vi "Dashboard Main.vi"() -> ()   [LabVIEW 2017]
uses:
  <vilib>/Utility/miscctls.llb/LVRowAndColumnTypeDef.ctl
  <vilib>/event_ctls.llb/eventvkey.ctl
  <vilib>/Rock Robotics/Network Tables/NT Read Numeric Array.vi
  <vilib>/Rock Robotics/WPI/Dashboard/WPI_DashboardLogging Global.vi
panel:
  out "Background 4":bool
  out "Background 3":bool
  out "Background 2":bool
  out "Background":bool
  in  "Camera Settings Right":T1={"Frame Rate"=30, "Compression"=30, "Size"=1, "DB Camera Config"=FALSE} {"Frame Rate" scale=1.0..30.0; "Compression" scale=100.0..-1.0; "Size" items=["640x480", "320x240", "160x120"]}
  in  "Camera Name Right":string(combo)="No Camera Selection"
  out "Camera Info":cluster{"Mbps LED":bool, "Mbps":dbl, "fps":dbl} {"fps" format="%#.1g"; "Mbps" format="%#.1g"}
  in  "Camera Settings":T1={"Frame Rate"=30, "Compression"=30, "Size"=1, "DB Camera Config"=FALSE} {"Frame Rate" scale=1.0..30.0; "Compression" scale=100.0..-1.0; "Size" items=["640x480", "320x240", "160x120"]}
  in  "TCP":refnum<k5>
  in  "Rec Mode":enum32{"Stop", "Record", "Playback"}(radio)
  out "Robot IP":string
  out "Image Message":string="Timeout in Camera Communications"
  in  "Dashboard Tab":T2(tab)
  out "Robot Lift Lower DIO3":bool
  out "Robot Lift Upper DIO2":bool
  out "Cube Lift DIO4":bool
  in  "Select Auto":string(combo)="Select Autonomous ..."
  out "NT Connection":bool
  out "MotorChart R":cluster{"Numeric":dbl, "Numeric":dbl}(graph)
  out "MotorChart L":cluster{"Numeric":dbl, "Numeric":dbl}(graph)
  out "MotorSliders R":cluster{"MotorSlide1":dbl, "MotorSlide2":dbl} {"MotorSlide2" scale=-1.0..1.0 scale format="%#_2e"; "MotorSlide1" scale=-1.0..1.0 scale format="%#_2e"}
  out "MotorSliders L":cluster{"MotorSlide1":dbl, "MotorSlide2":dbl} {"MotorSlide2" scale=-1.0..1.0 scale format="%#_2e"; "MotorSlide1" scale=-1.0..1.0 scale format="%#_2e"}
  out "Gyro":dbl(knob) scale=0.0..360.0
  out "JS1 Z":dbl(slide) scale=-1.0..1.0 scale format="%#_2e"
  out "JS1 Graph":cluster{"X":dbl, "Y":dbl}[](graph)
  out "JS1 Buttons":T3
  out "JS2 Z":dbl(slide) scale=-1.0..1.0 scale format="%#_2e"
  out "JS2 Graph":cluster{"X":dbl, "Y":dbl}[](graph)
  out "JS2 Buttons":T3
  out "Mode":T4(ring)=enum."Auto Disabled"
  out "Camera Image Right":T5(plugin-control)
  in  "Drive Style Selection":string(combo)="FPS"
  in  "Cube Intake Speed":dbl=10.0 min=0.0 max=10.0 step=1.0
  in  "H-Wheel":dbl=10.0 min=0.0 max=10.0 step=1.0
  in  "X-AXIS":dbl=10.0 min=0.0 max=10.0 step=1.0
  in  "Y-AXIS":dbl=10.0 min=0.0 max=10.0 step=1.0
  in  "Drive Motor Controller Selection":string(combo)="Talon SRX"
  in  "Cube Lift Down Speed":dbl=10.0 min=0.0 max=10.0 step=1.0
  in  "H-Wheel Motor Controller Selection":string(combo)="Spark"
  in  "Robot Lift Speed":dbl=10.0 min=0.0 max=10.0 step=1.0
  in  "Cube Lift Up Speed":dbl=10.0 min=0.0 max=10.0 step=1.0
  in  "MSR Slow Speed":dbl=0.5
  in  "MSR Slow Time":dbl=10.0
  in  "MSR Fast Speed":dbl=0.9
  in  "MSR Strafe Speed":dbl=0.6
  in  "MSR Fast Time":dbl=80.0
  in  "MSR Strafe Time":dbl=20.0
  in  "Move from Wall Speed":dbl=0.5
  in  "Move from Wall time":dbl=10.0
  in  "Strafe Speed":dbl=0.9
  in  "Forward Speed":dbl=0.6
  in  "Strafe Time":dbl=80.0
  in  "Forward Time":dbl=20.0
  in  "Test Slider":dbl(slide) scale=0.0..100.0 scale format="%#_3g"
  in  "On/Off":bool caption="Solenoid"
  in  "Test Name":u16(ring) items=["Select the test to run..."]
  in  "Test Tree":string(tree)
  in  "Motor":cluster{"Value":dbl, "Enable":bool} {"Value" scale=-1.0..1.0 scale format="%#_3g"}
  out "Progress":T6 {"Test Progress" scale=0.0..100.0}
  in  "Rev/Fwd":cluster{"Forward":bool, "Reverse":bool}
  in  "Test Ring":u16(ring) items=["Monochrome", "Color"]
  out "Cmd Status":string
  in  "Execute Command":bool
  in  "Command Params":string[][](table)
  in  "Command Selection":i32(listbox)
  in  "CheckList":i32(listbox)
  out "Tree":string(tree)
  out "Camera Image":T5(plugin-control)
  in  "Camera Name":string(combo)="No Camera Selection"
  # "HW"
  # "HW"
  # "Joysticks"
  # "Drive Motors"
  # "Front"
  # "Right"
  # "Left"
  # "Back"
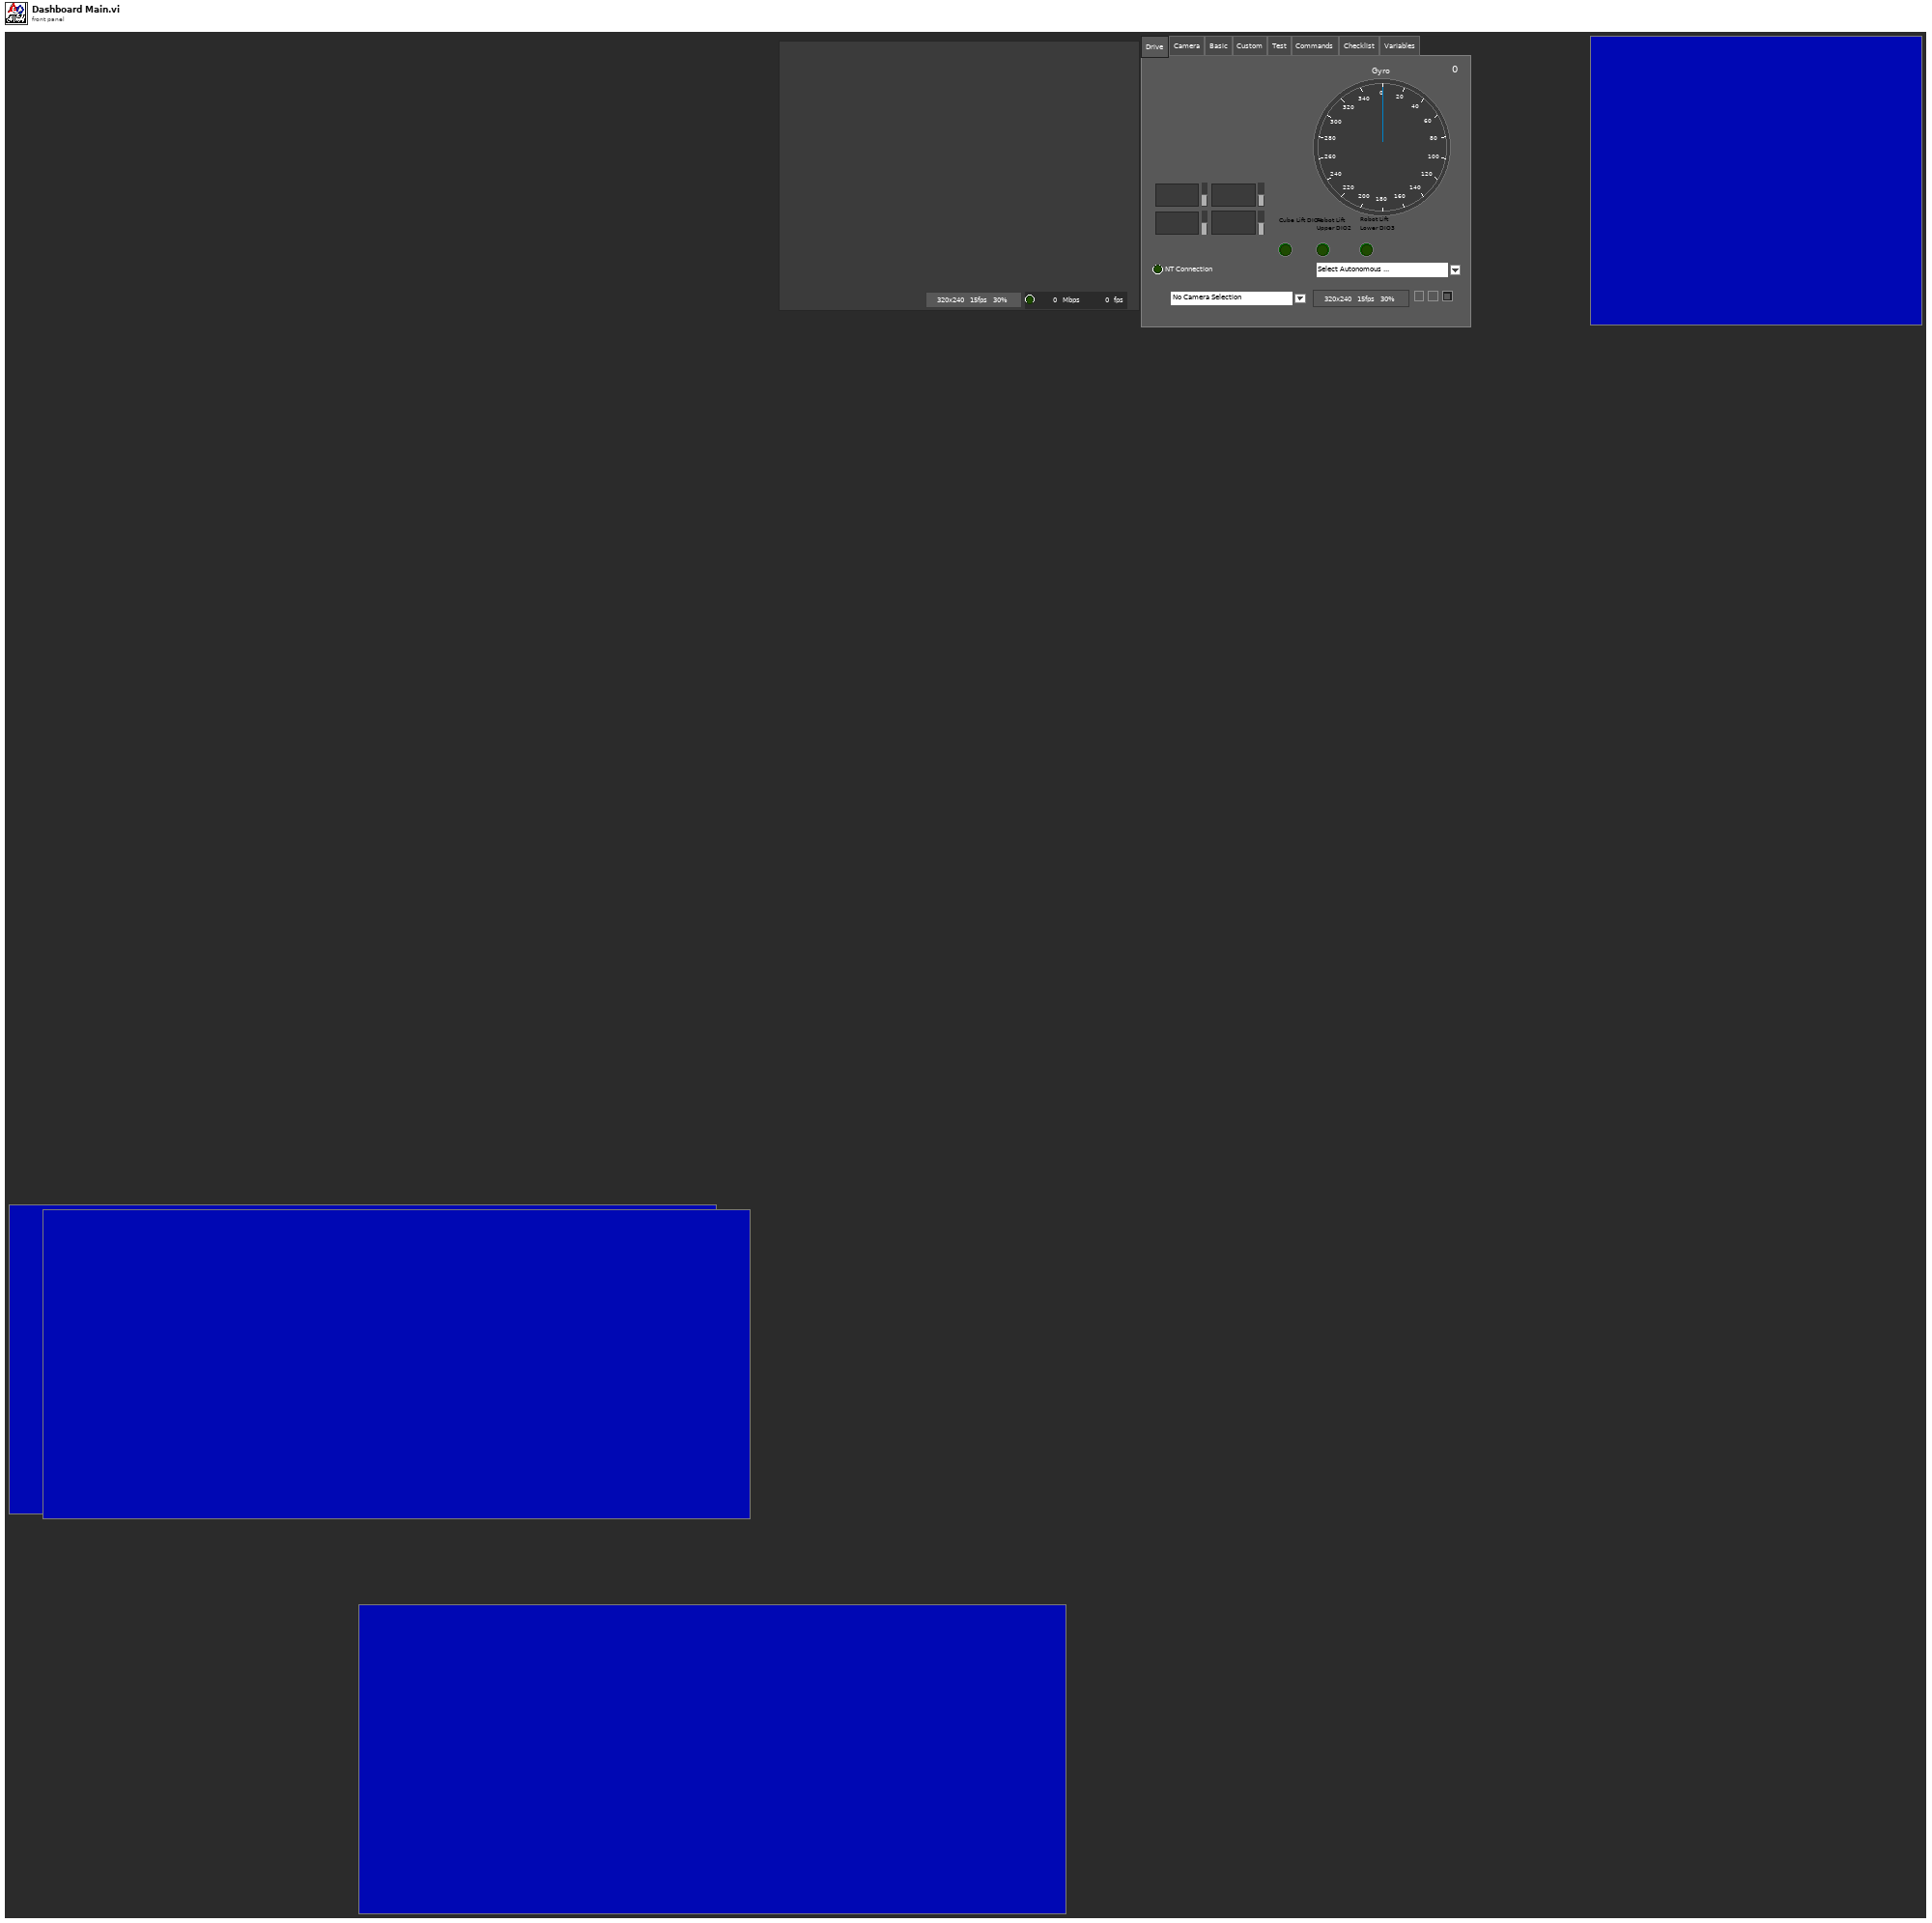
[diagram p1: front panel]
types:
  T1 = cluster{"Frame Rate":i32, "Compression":i32, "Size":u16, "DB Camera Config":bool}
  T2 = enum32{"Drive", "Camera", "Basic", "Custom", "Test", "Commands", "Checklist", "Variables"}
  T3 = cluster{bool, bool, bool, bool, bool, bool, bool, bool, bool, bool, bool, bool}
  T4 = enum8{"Tele-Op Disabled", "Tele-Op Enabled", "Auto Disabled", "Auto Enabled", "Test Disabled", "Test Enabled", "Disconnected", "No Code", "E-Stop"}
  T5 = typedef "IMAQ Image.ctl" = refnum<image>
  T6 = cluster{"Test Progress":u8, "Test Progress Text":string}
  T7 = cluster{"Save Path":path, "Interval (s)":dbl, "Keep":i32}
  T8 = typedef "Image Type" = u32
  T9 = cluster{"IDs":cluster{"RPC field ID":u16, "Unique ID":u16}, "String":string}
  T10 = cluster{"Error Strings":string, "Disable Counts":cluster{u16, u16}, "Rail Faults":cluster{u16, u16, u16}, "Robot IP":string, "DB Mode":u8, "Event Info":cluster{"Name":string, "Type":u8, "Number":u16, "Replay":u8}}
  T11 = cluster{"Storage":cluster{"Disk Free":u64, "RAM Block":u32, "RAM free":u32}, "CPU Utilization":cluster{"CPU % ISR":sgl, "CPU % Time Crit":sgl, "CPU % Timed Str":sgl, "CPU % High":sgl, "CPU % Above":sgl, "CPU % Normal":sgl, "CPU % Low":sgl}, "CAN":cluster{"% Bus Utilization":sgl, "Bus Off Cnt":u32, "TX_FIFO Full Cnt":u32, "Receive Error Cnt":u8, "Transmit Error Cnt":u8}, "HID":cluster{"HID Outputs":u32, "Rumble Low":u16, "Rumble High":u16}[]}
  T12 = cluster{"Status bits":cluster{"Test Mode":bool, "Autonomous":bool, "Enabled":bool, "Code Start":bool, "Brownout":bool, "Reserved 2":bool, "Reserved 3":bool, "E-Stop":bool}, "Code Trace":cluster{"Disabled":bool, "TeleOp":bool, "Auto":bool, "Test":bool}, "Controller Type":enum16{"unknown", "cRIO", "roboRio"}, "Code?":enum16{"unknown", "noCode", "code"}, "Battery V":dbl}
  T13 = cluster{"Control Bits":cluster{"TestMode":bool, "Autonomous":bool, "Enabled":bool, "FMS Present":bool, bool, bool, bool, "E-Stop":bool}, "Team Station ":u8, "Countdown":sgl, "Joystick Values":cluster{"Axes":dbl[], "Buttons":bool[], "POVs":i16[]}[]}
  T14 = cluster{"Axes":dbl[], "Buttons":bool[], "POVs":i16[]}[]
  T15 = cluster{"Axes":dbl[], "Buttons":bool[], "POVs":i16[]}
  T16 = cluster{"Buttons[0]":bool, "Buttons[1]":bool, "Buttons[2]":bool, "Buttons[3]":bool, "Buttons[4]":bool, "Buttons[5]":bool, "Buttons[6]":bool, "Buttons[7]":bool, "Buttons[8]":bool, "Buttons[9]":bool, "Buttons[10]":bool, "Buttons[11]":bool}
  T17 = cluster{"Camera Image":refnum<vi>, "Dashboard Tab":refnum<vi>, "Background 4":refnum<vi>, "Rec Mode":refnum<vi>, "Test Slider":refnum<vi>, "On/Off ":refnum<vi>, "Test Ring":refnum<vi>, "Rev/Fwd":refnum<vi>, "Test Name":refnum<vi>, "Motor":refnum<vi>, "Progress":refnum<vi>, "CheckList":refnum<vi>, "Tree":refnum<vi>, "Test Tree":refnum<vi>, "Command Params":refnum<vi>, "Command Selection":refnum<vi>, "Execute Command":refnum<vi>, "Cmd Status":refnum<vi>, "Camera Settings":refnum<vi>, "Camera Name":refnum<vi>, "Camera Info":refnum<vi>, "Camera Settings Right":refnum<vi>, "Camera Name Right":refnum<vi>, "Camera Image Right":refnum<vi>}
  T18 = cluster{"Camera Name":string, string, "Saved DB Images Info":cluster{"Save Path":path, "Interval (s)":dbl, "Keep":i32}}
  T19 = cluster{"Camera Name Right":string, string, "Saved DB Images Info":cluster{"Save Path":path, "Interval (s)":dbl, "Keep":i32}}
  T20 = cluster{"Operation":enum16{"Update", "Clear"}, "Color Box":u32}[]
  T21 = typedef "eventvkey.ctl" = enum16{"ASCII", "Enter", "Return", "Shift", "Ctrl", "Alt", "Cmd", "Opt", "Caps", "NumLock", "Clear", "Break", "Up", "Down", "Left", "Right", "Insert", "Delete", "Home", "End", "PageUp", "PageDown", "Escape", "Help", "Pause", "ScrollLock", "F1", "F2", "F3", "F4", "F5", "F6", "F7", "F8", "F9", "F10", "F11", "F12", "F13", "F14", "F15", "F16", "F17", "F18", "F19", "F20", "F21", "F22", "F23", "F24", "Play", "VolumeUp", "VolumeDown", "Mute", "Two Byte Char"}
  T22 = cluster{"Image Size":bool, "Image Type":bool, "Pixel Value":bool, "ROI Information":bool, "Zoom Factor":bool}
  T23 = cluster{"Operation":enum16{"Update", "Clear"}, "Color Box":u32}
  T24 = typedef "LVRowAndColumnTypeDef.ctl" = cluster{"Row":i32, "Column":i32}
  T25 = cluster{"Shift":bool, "Ctrl":bool, "Alt":bool, "Cmd":bool, "Opt":bool}
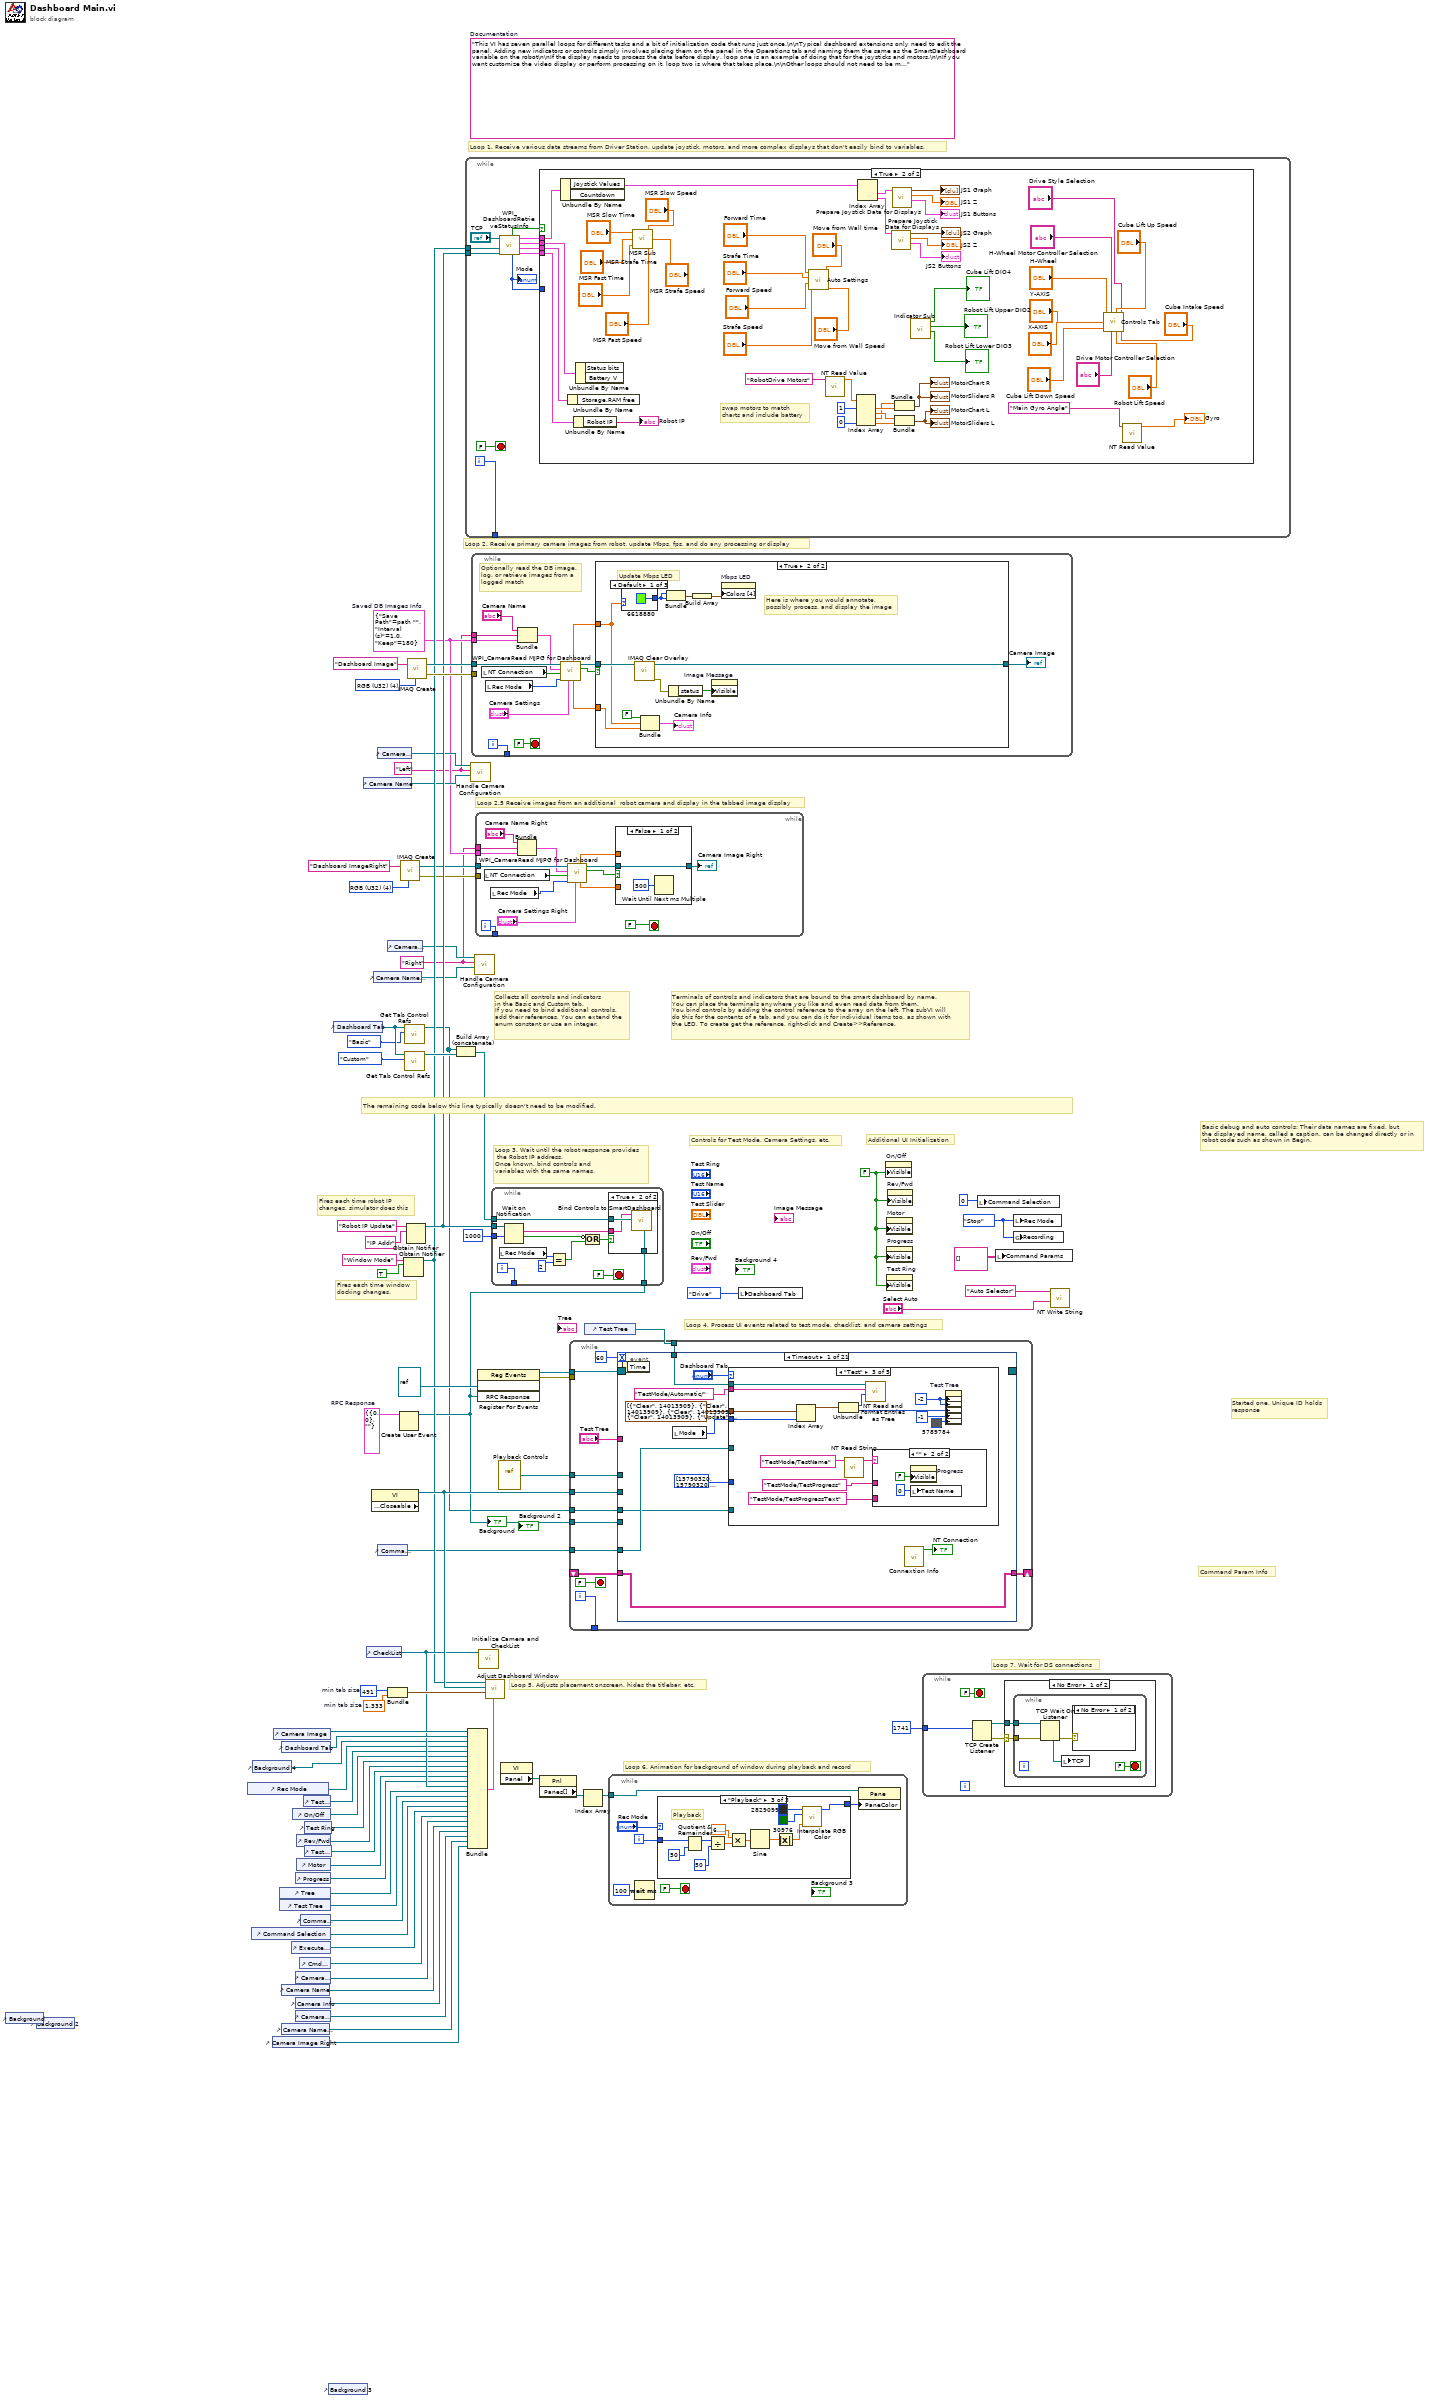
[diagram p0: block diagram]
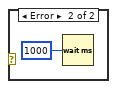
[diagram p3: hidden frame]
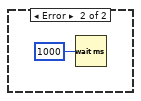
[diagram p4: hidden frame]
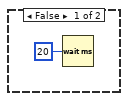
[diagram p5: hidden frame]
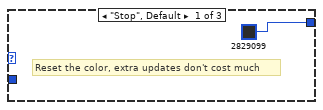
[diagram p6: hidden frame]
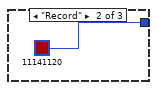
[diagram p7: hidden frame]
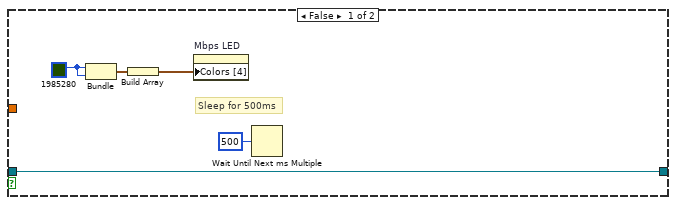
[diagram p9: hidden frame]
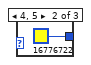
[diagram p10: hidden frame]
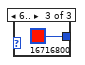
[diagram p11: hidden frame]
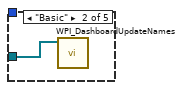
[diagram p13: hidden frame]
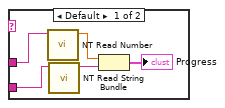
[diagram p14: hidden frame]
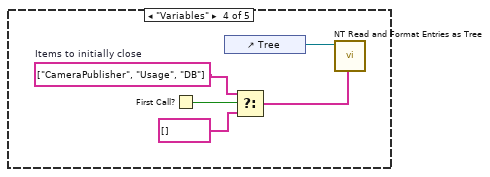
[diagram p15: hidden frame]
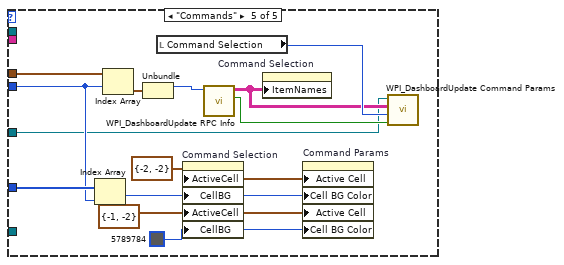
[diagram p16: hidden frame]
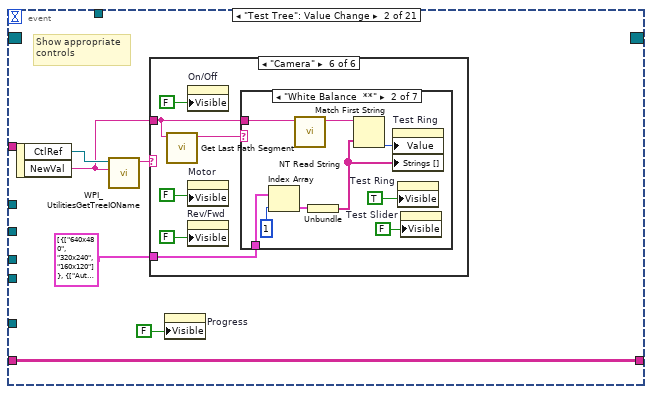
[diagram p17: hidden frame]
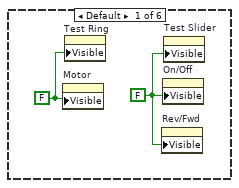
[diagram p18: hidden frame]
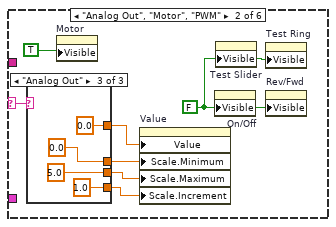
[diagram p19: hidden frame]
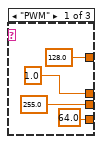
[diagram p20: hidden frame]
diagram:
  w4 = T7 {"Save Path"=path "", "Interval (s)"=1.0, "Keep"=180}  # Saved DB Images Info
  w3 = "Right"
  w2 = "Left"
  w14 = T8 4 items=["Grayscale (U8)", "Grayscale (I16)", "Grayscale (SGL)", "Complex (CSG)", "RGB (U32)", "HSL (U32)", "RGB (U64)"] ("Image Type")
  w30 = T9 {"IDs"={"RPC field ID"=0, "Unique ID"=0}, "String"=""}  # RPC Response
  w52 = 491  # min tab size
  w51 = 1.333  # min tab size
  w59 = enum32{"Stop", "Record", "Playback"}."Stop" ("Rec Mode")
  w37 = FALSE ("Visible")
  (unwired) "This VI has seven parallel loops for different tasks and a bit of initialization code that runs just once.\n\nTypical dashboard extensions only need to edit the panel. Adding new indicators or controls simply involves placing them on the panel in the Operations tab and naming them the same as the SmartDashboard variable on the robot\n\nIf the display needs to process the data before display, loop one is an example of doing that for the joysticks and motors.\n\nIf you want customize the video display or perform processing on it, loop two is where that takes place.\n\nOther loops should not need to be modified. They are pretty standard, and document the task they perform."  # Documentation
  w76 = T8 4 items=["Grayscale (U8)", "Grayscale (I16)", "Grayscale (SGL)", "Complex (CSG)", "RGB (U32)", "HSL (U32)", "RGB (U64)"] ("Image Type")
  # "Loop 2.5 Receive images from an additional  robot camera and display in the tabbed image display"
  # "Command Param Info"
  # "Started one, Unique ID holds\nresponse"
  # "Loop 7. Wait for DS connections"
  # "Basic debug and auto controls: Their data names are fixed, but\nthe displayed name, called a caption, can be changed directly or in\nrobot code such as shown in Begin."
  # "Controls for Test Mode, Camera Settings, etc."
  # "Additional UI Initialization"
  # "Loop 6. Animation for background of window during playback and record"
  # "Fires each time robot IP\nchanges, simulator does this"
  # "Fires each time window\ndocking changes."
  # "Collects all controls and indicators\nin the Basic and Custom tab.\nIf you need to bind additional controls,\nadd their references. You can extend the\nenum constant or use an integer."
  # "The remaining code below this line typically doesn't need to be modified."
  # "Loop 4. Process UI events related to test mode, checklist, and camera settings"
  # "Terminals of controls and indicators that are bound to the smart dashboard by name.\nYou can place the terminals anywhere you like and even read data from them.\nYou bind controls by adding the control reference to the array on the left. The subVI will\ndo this for the contents of a tab, and you can do it for individual items too, as shown with\nthe LED. To create get the reference, right-click and Create>>Reference."
  # "Loop 3. Wait until the robot response provides\n the Robot IP address.\nOnce known, bind controls and\nvariables with the same names."
  # "Loop 5. Adjusts placement onscreen, hides the titlebar, etc."
  # "Loop 1. Receive various data streams from Driver Station, update joystick, motors, and more complex displays that don't easily bind to variables."
  # "Loop 2. Receive primary camera images from robot, update Mbps, fps, and do any processing or display"
  n1 = control-ref of="Background"() -> ()  [unwired: 1 out]
  n2 = control-ref of="Background 2"() -> ()  [unwired: 1 out]
  n3 = control-ref of="Rec Mode"() -> (w43:refnum<vi>)
  n4 = control-ref of="Command Selection"() -> (w29:refnum<vi>)
  n5 = control-ref of="Background 4"() -> (w1:refnum<vi>)
  n6 = control-ref of="Camera Image Right"() -> (w7:refnum<vi>)
  n7 = control-ref of="Camera Image"() -> (w54:refnum<vi>)
  n8 = control-ref of="Tree"() -> (w47:refnum<vi>)
  n9 = control-ref of="Test Tree"() -> (w46:refnum<vi>)
  n10 = control-ref of="Dashboard Tab"() -> (w53:refnum<vi>)
  n11 = control-ref of="Camera Name"() -> (w20:refnum<vi>)
  n12 = control-ref of="Camera Name Right"() -> (w8:refnum<vi>)
  n13 = control-ref of="Execute Command"() -> (w31:refnum<vi>)
  n14 = control-ref of="On/Off"() -> (w41:refnum<vi>)
  n15 = control-ref of="Progress"() -> (w38:refnum<vi>)
  n16 = control-ref of="Camera Settings"() -> (w21:refnum<vi>)
  n17 = control-ref of="Camera Info"() -> (w19:refnum<vi>)
  n18 = control-ref of="Camera Settings Right"() -> (w9:refnum<vi>)
  n19 = control-ref of="Rev/Fwd"() -> (w39:refnum<vi>)
  n20 = control-ref of="Motor"() -> (w44:refnum<vi>)
  n21 = control-ref of="Cmd Status"() -> (w25:refnum<vi>)
  n22 = control-ref of="Command Params"() -> (w32:refnum<vi>)
  n23 = control-ref of="Test Slider"() -> (w42:refnum<vi>)
  n24 = control-ref of="Test Ring"() -> (w40:refnum<vi>)
  n25 = control-ref of="Test Name"() -> (w45:refnum<vi>)
  n26 = control-ref of="Background 3"() -> ()  [unwired: 1 out]
  n27 = control-ref of="Dashboard Tab"() -> (w57:refnum<vi>)
  n28 = control-ref of="Camera Name"() -> (w22:refnum<vi>)
  n29 = control-ref of="CheckList"() -> (w48:refnum<vi>)
  n30 = property class="VI" props=["Front Panel.Closeable"]() -> (reference out=w58:refnum<vi>)  [unwired: 2 in, 2 out]
  n31 = control-ref of="Camera Name Right"() -> (w10:refnum<vi>)
  n32 = control-ref of="Camera Settings"() -> (w23:refnum<vi>)
  n33 = control-ref of="Command Params"() -> (w24:refnum<vi>)
  n34 = control-ref of="Camera Settings Right"() -> (w11:refnum<vi>)
  n35 = Bundle("min tab size"=w52, "min tab size"=w51) -> (w50:cluster{"min tab size":i32, "min tab size":dbl})  [unwired: 1 in]
  n36 = Create User Event(user event datatype=w30) -> (user event=w26:refnum<user-event>)  [unwired: 1 in, 1 out]
  n37 = call "IMAQ Create"("Image Name"="Dashboard ImageRight", "Image Type"=w14) -> ("New Image"=w13:T5, "error out"=w12:errorcluster)  [unwired: 2 in, 1 out]
  n38 = Obtain Notifier(name (unnamed)="Window Mode", notification data type=TRUE) -> (notifier out=w35:refnum<notifier>)  [unwired: 2 in, 2 out]
  n39 = call <vilib>:"Get Tab Control Refs.vi"("Page Index"=T2."Basic" ("Dashboard Tab"), "TabControl in"=w57) -> ("ControlsOnPage"=w18:refnum<vi>[])  [unwired: 9 in]
  n40 = call <vilib>:"Get Tab Control Refs.vi"("Page Index"=T2."Custom" ("Dashboard Tab"), "TabControl in"=w57) -> ("ControlsOnPage"=w56:refnum<vi>[])  [unwired: 9 in]
  n41 = Obtain Notifier(name (unnamed)="Robot IP Update", notification data type="IP Addr" ("name (unnamed)")) -> (notifier out=w36:refnum<notifier>)  [unwired: 2 in, 2 out]
  n42 = call "IMAQ Create"("Image Name"="Dashboard Image", "Image Type"=w76) -> ("New Image"=w74:T5, "error out"=w73:errorcluster)  [unwired: 2 in, 1 out]
  n43 = Build Array (concatenate)(w18, w56) -> (w55:refnum<vi>[])
  n44 = while {
    tunnel: [w86] -> _
    tunnel: w36 -> [w80]
    tunnel: w35 -> [w77]
    i -> [w86]
    stop <- FALSE stop-if-true
    n45 = call <vilib>:"WPI_DashboardRetrieveStatusInfo.vi"("Binding Refnum"=w80, "Window Mode Notifier"=w77, "TCP Cnx"="TCP") -> ("Power and Errors"=w81:T10, "Robot Metrics"=w84:T11, "Status Info"=w85:T12, "Control Info"=w82:T13, "Robot Mode"=w79:T4, "Process?"=w83:bool)  [unwired: 3 in]
    "Mode" <- w79
    n46 = case shown="True" w83 {
      tunnel: w85 -> [_ w139]
      tunnel: w84 -> [_ w138]
      tunnel: w82 -> [_ w137]
      tunnel: w81 -> [_ w136]
      tunnel: w79 -> [_ _]
      frame False {
        n47 = Wait (ms)(milliseconds to wait=u32 20) -> ()  [unwired: 1 out]
      }
      frame True {
        # "swap motors to match\ncharts and include battery"
        n48 = Unbundle By Name(w137) -> ("Joystick Values"=w127:T14)  [unwired: 1 out]
        n49 = Unbundle By Name(w138) -> ()  [unwired: 1 out]
        n50 = Unbundle By Name(w136) -> ("Robot IP"=→"Robot IP":string)
        n51 = Unbundle By Name(w139) -> ()  [unwired: 2 out]
        n52 = call "MSR Sub.vi"("MSR Fast Speed"="MSR Fast Speed", "MSR Strafe Speed"="MSR Strafe Speed", "MSR Slow Speed"="MSR Slow Speed", "MSR Fast Time"="MSR Fast Time", "MSR Strafe Time"="MSR Strafe Time", "MSR Slow Time"="MSR Slow Time") -> ()
        n53 = call "Auto Settings.vi"("Mid Switch Forward Time"="Forward Time", "Mid Switch Strafe Time"="Strafe Time", "Mid Switch Forward Speed"="Forward Speed", "Mid Switch Strafe Speed"="Strafe Speed", "Strafe From Wall Time"="Move from Wall time", "Strafe From Wall Speed"="Move from Wall Speed") -> ()  [unwired: 5 in]
        n54 = call-poly <vilib>:"NT Read Value.vi"("Name"="RobotDrive Motors") -> ("Numeric Array"=w117:dbl[])  [unwired: 9 in, 1 out]
        n55 = Index Array(array=w117, index #1=1, index #4=0) -> (element #1=w131:dbl, element #2=w132:dbl, element #3=w130:dbl, element #4=w135:dbl)  [unwired: 2 in]
        n56 = Index Array(array=w127) -> (element #1=w126:T15, element #2=w122:T15)  [unwired: 2 in]
        n57 = call "Prepare Joystick Data for Displays.vi"("Joystick Values"=w122) -> ("Buttons"=→"JS2 Buttons":T16, "Z Axis"=→"JS2 Z":dbl, "Cartesian Data"=→"JS2 Graph":cluster{"X axis":dbl, "X axis":dbl}[])  [unwired: 8 in]
        n58 = call "Prepare Joystick Data for Displays.vi"("Joystick Values"=w126) -> ("Buttons"=→"JS1 Buttons":T16, "Z Axis"=→"JS1 Z":dbl, "Cartesian Data"=→"JS1 Graph":cluster{"X axis":dbl, "X axis":dbl}[])  [unwired: 8 in]
        n59 = Bundle("Numeric"=w130, "Numeric"=w131) -> (→"MotorChart R" →"MotorSliders R":cluster{"Numeric":dbl, "Numeric":dbl})  [unwired: 1 in]
        n60 = Bundle("Numeric"=w132, "Numeric"=w135) -> (→"MotorChart L" →"MotorSliders L":cluster{"Numeric":dbl, "Numeric":dbl})  [unwired: 1 in]
        n61 = call "Indicator Sub.vi"() -> ("Robot Lift Lower"=→"Robot Lift Lower DIO3":bool, "Robot Lift Upper"=→"Robot Lift Upper DIO2":bool, "Cube Lift"=→"Cube Lift DIO4":bool)  [unwired: 9 in]
        n62 = call "Controls Tab.vi"("H-Wheel"="H-Wheel", "H-Wheel Motor Controller Selection"="H-Wheel Motor Controller Selection", "Y-AXIS"="Y-AXIS", "Cube Lift Down Motor"="Cube Lift Down Speed", "Motor Controller Selection"="Drive Motor Controller Selection", "Cube Lift Up Motor"="Cube Lift Up Speed", "Drive Style Selection"="Drive Style Selection", "X-AXIS"="X-AXIS", "Robot Lift Motor"="Robot Lift Speed", "Cube Intake Motor"="Cube Intake Speed") -> ()
        n63 = call-poly <vilib>:"NT Read Value.vi"("Name"="Main Gyro Angle") -> ("Numeric"=→"Gyro":dbl)  [unwired: 9 in, 1 out]
      }
    }
  }
  n64 = Bundle("Camera Image"=w54, "Dashboard Tab"=w53, "Background 4"=w1, "Rec Mode"=w43, "Test Slider"=w42, "On/Off"=w41, "Test Ring"=w40, "Rev/Fwd"=w39, "Test Name"=w45, "Motor"=w44, "Progress"=w38, "CheckList"=w48, "Tree"=w47, "Test Tree"=w46, "Command Params"=w32, "Command Selection"=w29, "Execute Command"=w31, "Cmd Status"=w25, "Camera Settings"=w21, "Camera Name"=w20, "Camera Info"=w19, "Camera Settings Right"=w9, "Camera Name Right"=w8, "Camera Image Right"=w7) -> (w49:T17)  [unwired: 1 in]
  n65 = call "Handle Camera Configuration.vi"("CameraNameRef"=w22, "Display Name"=w2, "ClusterRef"=w23) -> ()  [unwired: 9 in]
  n66 = while {
    tunnel: w74 -> [w152]
    tunnel: w73 -> [_]
    tunnel: [w153] -> _
    tunnel: w4 -> [w143]
    tunnel: w2 -> [w140]
    i -> [w153]
    stop <- FALSE stop-if-true
    # "Optionally read the DB image,\nlog, or retrieve images from a\nlogged match"
    n67 = local read "NT Connection"() -> (w144:bool)
    n68 = local read "Rec Mode"() -> (w148:enum32{"Stop", "Record", "Playback"})
    n69 = Bundle("Camera Name"="Camera Name", w140, "Saved DB Images Info"=w143) -> (w142:T18)  [unwired: 1 in]
    n70 = call <vilib>:"WPI_CameraRead MJPG for Dashboard.vi"("Camera Settings"="Camera Settings", "Rec Mode"=w148, "NT Connection"=w144, "Capture Info"=w142, "Refnum in"=w152) -> ("Active"=w150:bool, "Refnum out"=w151:T5, "FPS"=w149:dbl, "Bandwidth (Mbps)"=w147:dbl)  [unwired: 3 in]
    n71 = case shown="True" w150 {
      tunnel: w151 -> [w155 w166]
      tunnel: w147 -> [_ w163]
      tunnel: w149 -> [_ w164]
      tunnel: [w155 w160] -> w145
      frame False {
        w157 = u32 1985280 ("Color Box")
        # "Sleep for 500ms"
        n72 = Bundle("Color Box"=w157, "Color Box"=w157) -> (w158:cluster{"Color Box":u32, "Color Box":u32})  [unwired: 1 out]
        n73 = Build Array(w158) -> (w156:cluster{"Color Box":u32, "Color Box":u32}[])
        n74 = property on="Mbps LED" class="Bool (strict)"("Colors [4]"=w156) -> ()  [unwired: 2 in, 2 out]
        n75 = Wait Until Next ms Multiple(millisecond multiple=u32 500) -> ()  [unwired: 1 out]
      }
      frame True {
        # "Here is where you would annotate,\npossibly process, and display the image"
        # "Update Mbps LED"
        n76 = case shown="Default" w163 {
          tunnel: [u32 6618880 ("Color Box") u32 16776722 ("Color Box") u32 16716800 ("Color Box")] -> w167
          frame Default {
          }
          frame 4, 5 {
          }
          frame 6.. {
          }
        }
        n77 = call "IMAQ Clear Overlay"("Image"=w166) -> ("error out"=w169:errorcluster, "Image Out"=w160:T5)  [unwired: 2 in, 7 out]
        n78 = Bundle(FALSE, "Bandwidth (Mbps)"=w163, "FPS"=w164) -> (→"Camera Info":cluster{bool, "Bandwidth (Mbps)":dbl, "FPS":dbl})  [unwired: 1 in]
        n79 = Bundle("Color Box"=w167, "Color Box"=w167) -> (w168:cluster{"Color Box":u32, "Color Box":u32})  [unwired: 1 out]
        n80 = Unbundle By Name(w169) -> ("status"=w170:bool)
        n81 = Build Array(w168) -> (w165:cluster{"Color Box":u32, "Color Box":u32}[])
        n82 = property on="Image Message" class="Str"("Visible"=w170) -> ()  [unwired: 2 in, 2 out]
        n83 = property on="Mbps LED" class="Bool (strict)"("Colors [4]"=w165) -> ()  [unwired: 2 in, 2 out]
      }
    }
    "Camera Image" <- w145
  }
  n84 = call "Handle Camera Configuration.vi"("CameraNameRef"=w10, "Display Name"=w3, "ClusterRef"=w11) -> ()  [unwired: 9 in]
  n85 = while {
    tunnel: w13 -> [w188]
    tunnel: w12 -> [_]
    tunnel: [w183] -> _
    tunnel: w4 -> [w177]
    tunnel: w3 -> [w174]
    i -> [w183]
    stop <- FALSE stop-if-true
    n86 = local read "NT Connection"() -> (w178:bool)
    n87 = local read "Rec Mode"() -> (w187:enum32{"Stop", "Record", "Playback"})
    n88 = Bundle("Camera Name Right"="Camera Name Right", w174, "Saved DB Images Info"=w177) -> (w176:T19)  [unwired: 1 in]
    n89 = call <vilib>:"WPI_CameraRead MJPG for Dashboard.vi"("Camera Settings"="Camera Settings Right", "Rec Mode"=w187, "NT Connection"=w178, "Capture Info"=w176, "Refnum in"=w188) -> ("Active"=w182:bool, "Refnum out"=w185:T5, "FPS"=w180:dbl, "Bandwidth (Mbps)"=w181:dbl)  [unwired: 3 in]
    n90 = case shown="False" w182 {
      tunnel: w185 -> [w189 w191]
      tunnel: w181 -> [_ _]
      tunnel: w180 -> [_ _]
      tunnel: [w189 w191] -> w179
      frame False {
        n91 = Wait Until Next ms Multiple(millisecond multiple=u32 500) -> ()  [unwired: 1 out]
      }
      frame True {
      }
    }
    "Camera Image Right" <- w179
  }
  n92 = register-events(refnum<vi> refnum, w26) -> (reference out=w63:refnum<event-registration>, error out=w62:errorcluster)  [unwired: 2 in]
  n93 = call "Initialize Camera and CheckList.vi"("ListBox in"=w48) -> ()  [unwired: 11 in]
  n94 = call "Adjust Dashboard Window.vi"("Sizing Refnums"=w49, "Size Constraints"=w50, "VI"=w58, "WIn Mode"=w35) -> ()  [unwired: 8 in]
  n95 = while {
    tunnel: w55 -> [w203]
    tunnel: w36 -> [w201]
    tunnel: [w199] -> _
    tunnel: u32 1000 ("milliseconds to wait") -> [w198]
    tunnel: w26 -> [w192]
    i -> [w199]
    stop <- FALSE stop-if-true
    n96 = local read "Rec Mode"() -> (w194:enum32{"Stop", "Record", "Playback"})
    n97 = Wait on Notification(notifier=w201, timeout in ms (-1)=w198) -> (notification=w200:string, timed out?=w196:bool)  [unwired: 2 in, 2 out]
    n98 = Equal?(x=w194, y=u16 2 ("Rec Mode")) -> (x = y?=w195:bool)
    n99 = Compound Arithmetic op=OR(invert w196, w195) -> (w197:bool)
    n100 = case shown="True" w197 {
      tunnel: w203 -> [_ w206]
      tunnel: w200 -> [_ w205]
      tunnel: w192 -> [_ w204]
      frame False {
      }
      frame True {
        n101 = call <vilib>:"Bind Controls to SmartDashboard.vi"("RPC ref"=w204, "Bound Control Refs"=w206, "Server IP Address"=w205) -> ()  [unwired: 9 in]
      }
    }
  }
  n102 = vi-ref "Playback Controls.vi"() -> (w64:refnum<vi>)
  n103 = property class="VI"() -> ("Panel"=w66:refnum<vi>)  [unwired: 2 in, 2 out]
  n104 = property class="Pnl"(reference=w66) -> ("Panes[]"=w67:refnum<vi>[])  [unwired: 1 in, 2 out]
  n105 = Index Array(array=w67) -> (element=w65:refnum<vi>)  [unwired: 1 in]
  n106 = control-ref of="Test Tree"() -> (w68:refnum<vi>)
  n107 = while {
    tunnel: [w216] -> _
    tunnel: w68 -> [w215]
    tunnel: w64 -> [w214]
    tunnel: w63 -> [w213]
    tunnel: w62 -> [_]
    tunnel: w58 -> [w212]
    tunnel: w26 -> [w211]
    tunnel: w24 -> [w210]
    shift-right: [w209] -> _
    shift-left: _ -> [w208]
    tunnel: w18 -> [w207]
    i -> [w216]
    stop <- FALSE stop-if-true
    n108 = event shown="[0] Timeout" {
      selector: w213 -> [_ _ _ _ _ _ _ _ _ _ _ _ _ _ _ _ _ _ _ _ _]
      dyn-events: [_ _ _ _ _ _ _ _ _ _ _ _ _ _ _ _ w476 _ _ _ _] -> _
      timeout: u32 60 ("milliseconds to wait") -> [_ _ _ _ _ _ _ _ _ _ _ _ _ _ _ _ _ _ _ _ _]
      tunnel: w215 -> [w228 _ _ _ _ _ _ _ _ _ _ _ _ _ _ _ _ _ _ _ _]
      tunnel: "Test Tree" -> [_ _ _ _ _ _ _ _ _ _ _ w443 w451 w453 w457 w465 _ _ _ _ _]
      tunnel: w214 -> [_ _ _ _ _ _ _ _ _ _ _ _ _ _ _ _ w478 _ w496 _ _]
      tunnel: w212 -> [_ _ _ _ _ _ _ _ _ _ _ _ _ _ _ _ w474 _ _ _ _]
      tunnel: w211 -> [_ _ _ _ _ _ _ _ _ _ _ _ _ _ _ _ w472 _ _ _ _]
      tunnel: w210 -> [w223 _ _ _ _ _ w394 _ _ _ _ _ _ _ _ _ _ _ _ _ _]
      tunnel: [w222 w271 w373 w378 w387 w391 w392 w401 w411 w418 w430 w442 w449 w452 w456 w464 w471 w491 w493 w497 w510] -> w209
      tunnel: w208 -> [w222 w271 w373 w378 w387 w391 w392 _ _ w418 w430 w442 w449 w452 w456 w464 w471 w491 w493 w497 w510]
      tunnel: w207 -> [w220 _ _ _ _ _ _ _ _ _ _ _ _ _ _ _ _ _ _ _ _]
      event Timeout {
        n109 = event-data() -> ()  [unwired: 1 in, 1 out]
        n110 = local read "Mode"() -> (w225:T4)
        n111 = case shown="\"Test\"" "Dashboard Tab" {
          tunnel: w228 -> [_ _ w244 _ _]
          tunnel: "TestMode/Automatic/" ("Name Pattern") -> [_ _ w243 _ _]
          tunnel: T20 [{"Operation"=enum."Clear", "Color Box"=14013909}, {"Operation"=enum."Clear", "Color Box"=14013909}, {"Operation"=enum."Clear", "Color Box"=14013909}, {"Operation"=enum."Clear", "Color Box"=14013909}, {"Operation"=enum."Update", "Color Box"=14013909}, {"Operation"=enum."Update", "Color Box"=16777215}, {"Operation"=enum."Clear", "Color Box"=14013909}, {"Operation"=enum."Clear", "Color Box"=14013909}, {"Operation"=enum."Clear", "Color Box"=14013909}] -> [_ _ w236 _ w264]
          tunnel: w225 -> [_ _ w235 _ w263]
          tunnel: u32[] [15790320, 15790320, 15790320, 15790320, 16777215, 16777215, 15790320, 15790320, 15790320] -> [_ _ _ _ w269]
          tunnel: w223 -> [_ _ _ _ w257]
          tunnel: w220 -> [_ w230 _ _ _]
          frame "Custom", Default {
          }
          frame "Basic" {
            n112 = call <vilib>:"WPI_DashboardUpdateNames.vi"("Controls on Tab"=w230) -> ()  [unwired: 11 in]
          }
          frame "Test" {
            w242 = -2 ("Active Item:Row Number")
            n113 = Index Array(array=w236, index=w235) -> (element=w237:T23)
            n114 = Unbundle(w237) -> ("Operation"=w238:enum16{"Update", "Clear"}, "Color Box"=w239:u32)
            n115 = call <vilib>:"NT Read String.vi"("Name"="TestMode/TestName") -> ("String"=w233:string)  [unwired: 9 in, 1 out]
            n116 = call <vilib>:"NT Read and Format Entries as Tree.vi"("Operation"=w238, "Name Pattern"=w243, "Tree Refnum"=w244) -> ()  [unwired: 7 in, 2 out]
            n117 = case shown="\"\"" w233 {
              tunnel: "TestMode/TestProgress" ("Name") -> [w246 _]
              tunnel: "TestMode/TestProgressText" ("Name") -> [w245 _]
              frame Default {
                n118 = call <vilib>:"NT Read Number.vi"("Name"=w246) -> ("Numeric"=w247:dbl)  [unwired: 9 in, 1 out]
                n119 = call <vilib>:"NT Read String.vi"("Name"=w245) -> ("String"=w248:string)  [unwired: 9 in, 1 out]
                n120 = Bundle("Numeric"=w247, "String"=w248) -> (→"Progress":cluster{"Numeric":dbl, "String":string})  [unwired: 1 in]
              }
              frame "" {
                n121 = property on="Progress" class="Clust (strict)"("Visible"=FALSE) -> ()  [unwired: 2 in, 2 out]
                n122 = local write "Test Name"(u16 0) -> ()
              }
            }
            n123 = property on="Test Tree" class="Tree (strict)"("Active Item Row Number"=w242, "ActiveColNum"=w242, "CellBG"=w239, "Active Item Row Number"=-1 ("Active Item:Row Number"), "CellBG"=u32 5789784 ("Color Box")) -> ()  [unwired: 2 in, 2 out]
          }
          frame "Variables" {
            w254 = string[] ["CameraPublisher", "Usage", "DB"]  # Items to initially close
            n124 = First Call?() -> (First Call?: T/F=w255:bool)
            n125 = control-ref of="Tree"() -> (w256:refnum<vi>)
            n126 = Select(t=w254, s=w255, f=string[] []) -> (s? t:f=w252:string[])
            n127 = call <vilib>:"NT Read and Format Entries as Tree.vi"("Tags to  Close"=w252, "Tree Refnum"=w256) -> ()  [unwired: 8 in, 2 out]
          }
          frame "Commands" {
            w265 = u32 5789784 ("Color Box")
            w266 = T24 {"Row"=-1, "Column"=-2} ("Active Cell:Active Cell")
            w268 = T24 {"Row"=-2, "Column"=-2} ("Active Cell:Active Cell")
            n128 = Index Array(array=w269, index=w263) -> (element=w267:u32)
            n129 = Index Array(array=w264, index=w263) -> (element=w262:T23)
            n130 = Unbundle(w262) -> ("Operation"=w261:enum16{"Update", "Clear"})  [unwired: 1 out]
            n131 = local read "Command Selection"() -> (w260:i32)
            n132 = property on="Command Selection" class="MCListbox (strict)"("ActiveCell"=w268, "CellBG"=w267, "ActiveCell"=w266, "CellBG"=w265) -> ()  [unwired: 2 in, 2 out]
            n133 = call <vilib>:"WPI_DashboardUpdate RPC Info.vi"("Operation"=w261) -> ("update"=w259:bool, "commands"=w258:string[][])  [unwired: 9 in]
            n134 = property on="Command Selection" class="MCListbox (strict)"("ItemNames"=w258) -> ()  [unwired: 2 in, 2 out]
            n135 = property on="Command Params" class="Tbl (strict)"("Active Cell"=w268, "Cell BG Color"=w267, "Active Cell"=w266, "Cell BG Color"=w265) -> ()  [unwired: 2 in, 2 out]
            n136 = call <vilib>:"WPI_DashboardUpdate Command Params.vi"("Update"=w259, "NewVal"=w260, "Commands"=w258, "Param Tbl"=w257) -> ()  [unwired: 7 in, 1 out]
          }
        }
        n137 = call <vilib>:"Connextion Info.vi"() -> ("Connected"=→"NT Connection":bool)  [unwired: 10 in, 1 out]
      }
      event "Test Tree": Value Change {
        # "Show appropriate\ncontrols"
        n138 = event-data() -> ("CtlRef"=w274:refnum<vi>, "NewVal"=w272:string)  [unwired: 1 in]
        n139 = call <vilib>:"WPI_UtilitiesGetTreeIOName.vi"("NewVal"=w272, "TreeControl in"=w274) -> ("I/O Name"=w275:string)  [unwired: 9 in]
        n140 = case shown="\"Camera\"" w275 {
          selector: w275 -> [_ w282 _ w304 w313 _]
          tunnel: w272 -> [_ _ w301 w303 _ w320]
          tunnel: cluster{string[]}[] [{["640x480", "320x240", "160x120"]}, {["Auto", "Fixed indoor", "Fixed outdoor 1", "Fixed outdoor 2", "Fixed fluorescent 1", "Fixed fluorescent 2", "Hold current"]}, {["Auto", "Flicker-free 50 Hz", "Flicker-free 60 Hz", "Hold current"]}, {["None", "Prioritize frame rate", "Prioritize image quality"]}, {["Monochrome", "Color"]}] -> [_ _ _ _ _ w319]
          frame Default {
            w277 = FALSE ("Visible")
            w276 = FALSE ("Visible")
            n141 = property on="Motor" class="Clust (strict)"("Visible"=w276) -> ()  [unwired: 2 in, 2 out]
            n142 = property on="Test Ring" class="Ring (strict)"("Visible"=w276) -> ()  [unwired: 2 in, 2 out]
            n143 = property on="Rev/Fwd" class="Clust (strict)"("Visible"=w277) -> ()  [unwired: 2 in, 2 out]
            n144 = property on="On/Off" class="Bool (strict)"("Visible"=w277) -> ()  [unwired: 2 in, 2 out]
            n145 = property on="Test Slider" class="Slide (strict)"("Visible"=w277) -> ()  [unwired: 2 in, 2 out]
          }
          frame "Analog Out", "Motor", "PWM" {
            w283 = FALSE ("Visible")
            n146 = case shown="\"Analog Out\"" w282 {
              tunnel: [1.0 ("Value") -1.0 ("Value") 0.0 ("Value")] -> w281
              tunnel: [255.0 ("Value") 1.0 ("Value") 5.0 ("Value")] -> w280
              tunnel: [128.0 ("Value") 0.0 ("Value") 0.0 ("Value")] -> w279
              tunnel: [64.0 ("Value") 0.5 ("Value") 1.0 ("Value")] -> w278
              frame "PWM" {
              }
              frame "Motor", Default {
              }
              frame "Analog Out" {
              }
            }
            n147 = property on="Motor" class="Clust (strict)"("Visible"=TRUE) -> ()  [unwired: 2 in, 2 out]
            n148 = property on="Value" class="Slide (strict)"("Value"=w279, "Scale.Minimum"=w281, "Scale.Maximum"=w280, "Scale.Increment"=w278) -> ()  [unwired: 2 in, 2 out]
            n149 = property on="On/Off" class="Bool (strict)"("Visible"=w283) -> ()  [unwired: 2 in, 2 out]
            n150 = property on="Test Slider" class="Slide (strict)"("Visible"=w283) -> ()  [unwired: 2 in, 2 out]
            n151 = property on="Test Ring" class="Ring (strict)"("Visible"=w283) -> ()  [unwired: 2 in, 2 out]
            n152 = property on="Rev/Fwd" class="Clust (strict)"("Visible"=w283) -> ()  [unwired: 2 in, 2 out]
          }
          frame "Servo" {
            w299 = FALSE ("Visible")
            n153 = call <vilib>:"NT Read Number.vi"("Name"=w301) -> ("Numeric"=w300:dbl)  [unwired: 9 in, 1 out]
            n154 = property on="Test Slider" class="Slide (strict)"("Visible"=TRUE, "Scale.Maximum"=170.0 ("Scale.Range:Maximum")) -> ()  [unwired: 2 in, 2 out]
            n155 = local write "Test Slider"(w300) -> ()
            n156 = property on="Motor" class="Clust (strict)"("Visible"=w299) -> ()  [unwired: 2 in, 2 out]
            n157 = property on="Rev/Fwd" class="Clust (strict)"("Visible"=w299) -> ()  [unwired: 2 in, 2 out]
            n158 = property on="On/Off" class="Bool (strict)"("Visible"=w299) -> ()  [unwired: 2 in, 2 out]
            n159 = property on="Test Ring" class="Ring (strict)"("Visible"=w299) -> ()  [unwired: 2 in, 2 out]
          }
          frame "Relay", "Solenoid" {
            w302 = FALSE ("Visible")
            n160 = property on="Motor" class="Clust (strict)"("Visible"=w302) -> ()  [unwired: 2 in, 2 out]
            n161 = property on="Test Slider" class="Slide (strict)"("Visible"=w302) -> ()  [unwired: 2 in, 2 out]
            n162 = Search and Replace String(input string=w303, search string="/Value  **", replace string="/Direction") -> (result string=w309:string)  [unwired: 5 in, 3 out]
            n163 = property on="Test Ring" class="Ring (strict)"("Visible"=w302) -> ()  [unwired: 2 in, 2 out]
            n164 = call <vilib>:"NT Read String.vi"("Name"=w309) -> ("String"=w307:string)  [unwired: 9 in, 1 out]
            n165 = Equal?(x="Both directions", y=w307) -> (x = y?=w305:bool)
            n166 = Not(x=w305) -> (.not. x?=w306:bool)
            n167 = property on="Rev/Fwd" class="Clust (strict)"("Visible"=w305) -> ()  [unwired: 2 in, 2 out]
            n168 = property on="On/Off" class="Bool (strict)"("Visible"=w306, "Caption.Text"=w304) -> ()  [unwired: 2 in, 2 out]
          }
          frame "Compressor", "Digital Out" {
            w312 = FALSE ("Visible")
            # "Get direction and finish"
            n169 = property on="Motor" class="Clust (strict)"("Visible"=w312) -> ()  [unwired: 2 in, 2 out]
            n170 = property on="Test Slider" class="Slide (strict)"("Visible"=w312) -> ()  [unwired: 2 in, 2 out]
            n171 = property on="Test Ring" class="Ring (strict)"("Visible"=w312) -> ()  [unwired: 2 in, 2 out]
            n172 = property on="On/Off" class="Bool (strict)"("Visible"=TRUE, "Caption.Text"=w313) -> ()  [unwired: 2 in, 2 out]
            n173 = property on="Rev/Fwd" class="Clust (strict)"("Visible"=FALSE) -> ()  [unwired: 2 in, 2 out]
          }
          frame "Camera" {
            n174 = call <vilib>:"Get Last Path Segment.vi"("String in"=w320) -> ("String out"=w321:string)  [unwired: 10 in]
            n175 = property on="On/Off" class="Bool (strict)"("Visible"=FALSE) -> ()  [unwired: 2 in, 2 out]
            n176 = property on="Motor" class="Clust (strict)"("Visible"=FALSE) -> ()  [unwired: 2 in, 2 out]
            n177 = property on="Rev/Fwd" class="Clust (strict)"("Visible"=FALSE) -> ()  [unwired: 2 in, 2 out]
            n178 = case shown="\"White Balance  **\"" w321 {
              tunnel: w320 -> [w327 w336 w345 w354 w363 _ w369]
              tunnel: w319 -> [w325 w333 w342 w351 w360 _ _]
              frame "Size  **" {
                n179 = Index Array(array=w325) -> (element=w324:cluster{string[]})  [unwired: 1 in]
                n180 = call <vilib>:"NT Read String.vi"("Name"=w327) -> ("String"=w326:string)  [unwired: 9 in, 1 out]
                n181 = Unbundle(w324) -> (w322:string[])
                n182 = Match First String(2:w322, 3:w326) -> (0:w323:i32)  [unwired: 1 out]
                n183 = property on="Test Ring" class="Ring (strict)"("Value"=w323, "Strings []"=w322) -> ()  [unwired: 2 in, 2 out]
                n184 = property on="Test Ring" class="Ring (strict)"("Visible"=TRUE) -> ()  [unwired: 2 in, 2 out]
                n185 = property on="Test Slider" class="Slide (strict)"("Visible"=FALSE) -> ()  [unwired: 2 in, 2 out]
              }
              frame "White Balance  **" {
                n186 = Index Array(array=w333, index=1) -> (element=w334:cluster{string[]})
                n187 = call <vilib>:"NT Read String.vi"("Name"=w336) -> ("String"=w335:string)  [unwired: 9 in, 1 out]
                n188 = Unbundle(w334) -> (w331:string[])
                n189 = Match First String(2:w331, 3:w335) -> (0:w330:i32)  [unwired: 1 out]
                n190 = property on="Test Ring" class="Ring (strict)"("Value"=w330, "Strings []"=w331) -> ()  [unwired: 2 in, 2 out]
                n191 = property on="Test Ring" class="Ring (strict)"("Visible"=TRUE) -> ()  [unwired: 2 in, 2 out]
                n192 = property on="Test Slider" class="Slide (strict)"("Visible"=FALSE) -> ()  [unwired: 2 in, 2 out]
              }
              frame "Exposure  **" {
                n193 = Index Array(array=w342, index=2) -> (element=w343:cluster{string[]})
                n194 = call <vilib>:"NT Read String.vi"("Name"=w345) -> ("String"=w344:string)  [unwired: 9 in, 1 out]
                n195 = Unbundle(w343) -> (w339:string[])
                n196 = Match First String(2:w339, 3:w344) -> (0:w340:i32)  [unwired: 1 out]
                n197 = property on="Test Ring" class="Ring (strict)"("Value"=w340, "Strings []"=w339) -> ()  [unwired: 2 in, 2 out]
                n198 = property on="Test Ring" class="Ring (strict)"("Visible"=TRUE) -> ()  [unwired: 2 in, 2 out]
                n199 = property on="Test Slider" class="Slide (strict)"("Visible"=FALSE) -> ()  [unwired: 2 in, 2 out]
              }
              frame "Exposure Priority  **" {
                n200 = Index Array(array=w351, index=3) -> (element=w352:cluster{string[]})
                n201 = call <vilib>:"NT Read String.vi"("Name"=w354) -> ("String"=w353:string)  [unwired: 9 in, 1 out]
                n202 = Unbundle(w352) -> (w348:string[])
                n203 = Match First String(2:w348, 3:w353) -> (0:w349:i32)  [unwired: 1 out]
                n204 = property on="Test Ring" class="Ring (strict)"("Value"=w349, "Strings []"=w348) -> ()  [unwired: 2 in, 2 out]
                n205 = property on="Test Ring" class="Ring (strict)"("Visible"=TRUE) -> ()  [unwired: 2 in, 2 out]
                n206 = property on="Test Slider" class="Slide (strict)"("Visible"=FALSE) -> ()  [unwired: 2 in, 2 out]
              }
              frame "Color Enable  **" {
                n207 = Index Array(array=w360, index=4) -> (element=w361:cluster{string[]})
                n208 = call <vilib>:"NT Read String.vi"("Name"=w363) -> ("String"=w362:string)  [unwired: 9 in, 1 out]
                n209 = Unbundle(w361) -> (w357:string[])
                n210 = Match First String(2:w357, 3:w362) -> (0:w358:i32)  [unwired: 1 out]
                n211 = property on="Test Ring" class="Ring (strict)"("Value"=w358, "Strings []"=w357) -> ()  [unwired: 2 in, 2 out]
                n212 = property on="Test Ring" class="Ring (strict)"("Visible"=TRUE) -> ()  [unwired: 2 in, 2 out]
                n213 = property on="Test Slider" class="Slide (strict)"("Visible"=FALSE) -> ()  [unwired: 2 in, 2 out]
              }
              frame Default {
                n214 = property on="Test Ring" class="Ring (strict)"("Visible"=FALSE) -> ()  [unwired: 2 in, 2 out]
                n215 = property on="Test Slider" class="Slide (strict)"("Visible"=FALSE) -> ()  [unwired: 2 in, 2 out]
              }
              frame "Brightness  **", "Color Level  **", "Compression  **", "FPS  **", "Sharpness  **" {
                n216 = call <vilib>:"NT Read Number.vi"("Name"=w369) -> ("Numeric"=w368:dbl)  [unwired: 9 in, 1 out]
                n217 = local write "Test Slider"(w368) -> ()
                n218 = property on="Test Slider" class="Slide (strict)"("Visible"=TRUE, "Scale.Maximum"=100.0 ("Scale.Range:Maximum")) -> ()  [unwired: 2 in, 2 out]
                n219 = property on="Test Ring" class="Ring (strict)"("Visible"=FALSE) -> ()  [unwired: 2 in, 2 out]
              }
            }
          }
        }
        n220 = property on="Progress" class="Clust (strict)"("Visible"=FALSE) -> ()  [unwired: 2 in, 2 out]
      }
      event "Test Name": Mouse Enter {
        # "Populate the ring with the list of tests"
        n221 = event-data() -> ()  [unwired: 1 in, 1 out]
        n222 = call <vilib>:"NT Read String Array.vi"("Name"="TestMode/TestList") -> ("String Array"=w377:string[])  [unwired: 9 in, 1 out]
        n223 = Build Array (concatenate)("Select the test to run...", w377) -> (w376:string[])
        n224 = property on="Test Name" class="Ring (strict)"("Strings []"=w376) -> ()  [unwired: 2 in, 2 out]
      }
      event "Test Name": Value Change {
        w379 = FALSE ("Visible")
        # "Tell the robot the test name to run"
        n225 = event-data() -> ("NewVal"=w383:u16)  [unwired: 1 in]
        n226 = property on="Test Name" class="Ring (strict)"() -> ("Strings []"=w384:string[])  [unwired: 2 in, 2 out]
        n227 = local write "Progress"(T6 {"Test Progress"=0, "Test Progress Text"=""} ("Progress")) -> ()
        n228 = Index Array(array=w384, index=w383) -> (element=w382:string)
        n229 = call <vilib>:"NT Write String.vi"("String"=w382, "Name"="TestMode/TestName") -> ()  [unwired: 9 in, 1 out]
        n230 = property on="Progress" class="Clust (strict)"("Visible"=TRUE) -> ()  [unwired: 2 in, 2 out]
        n231 = property on="Motor" class="Clust (strict)"("Visible"=w379) -> ()  [unwired: 2 in, 2 out]
        n232 = property on="Test Slider" class="Slide (strict)"("Visible"=w379) -> ()  [unwired: 2 in, 2 out]
        n233 = property on="On/Off" class="Bool (strict)"("Visible"=w379) -> ()  [unwired: 2 in, 2 out]
        n234 = property on="Rev/Fwd" class="Clust (strict)"("Visible"=w379) -> ()  [unwired: 2 in, 2 out]
        n235 = property on="Test Ring" class="Ring (strict)"("Visible"=w379) -> ()  [unwired: 2 in, 2 out]
      }
      event "Select Auto": Mouse Enter {
        # "Populate the combo box with the list of autonomous options"
        n236 = event-data() -> ()  [unwired: 1 in, 1 out]
        n237 = call <vilib>:"NT Read String Array.vi"("Name"="Auto List") -> ("String Array"=w386:string[])  [unwired: 9 in, 1 out]
        n238 = property on="Select Auto" class="CmbBox"("Strings[]"=w386) -> ()  [unwired: 2 in, 2 out]
      }
      event "Select Auto": Value Change {
        # "User modified the Auto Selection. Write to NT variable so robot knows."
        n239 = event-data() -> ("NewVal"=w389:string)  [unwired: 1 in]
        n240 = call <vilib>:"NT Write String.vi"("String"=w389, "Name"="Auto Selector") -> ()  [unwired: 9 in, 1 out]
      }
      event "Command Selection": Value Change {
        # "Get the params and show in table"
        n241 = event-data() -> ("NewVal"=w395:i32)  [unwired: 1 in]
        n242 = property on="Command Selection" class="MCListbox (strict)"() -> ("ItemNames"=w393:string[][])  [unwired: 2 in, 2 out]
        n243 = call <vilib>:"WPI_DashboardUpdate Command Params.vi"("NewVal"=w395, "Commands"=w393, "Param Tbl"=w394) -> ()  [unwired: 8 in, 1 out]
      }
      event "Execute Command": Value Change {
        # "Started one, Unique ID holds\nresponse"
        n244 = event-data() -> ()  [unwired: 1 in, 1 out]
        n245 = property on="Command Selection" class="MCListbox (strict)"() -> ("ItemNames"=w406:string[][])  [unwired: 2 in, 2 out]
        n246 = Index Array(array=w406, index (row)="Command Selection", index (col)=0) -> (element=w404:string)
        n247 = call <vilib>:"Invoke Commands.vi"("Command Params"="Command Params", "Function Name"=w404) -> ("Params"=w400:u8, "Started"=w399:bool)  [unwired: 7 in, 1 out]
        n248 = Array Subset(array="Command Params", length (row)=w400) -> (w401:string[][])  [unwired: 3 in]
        n249 = Select(t="Executing" ("Cmd Status"), s=w399, f="" ("Cmd Status")) -> (s? t:f=→"Cmd Status":string)
      }
      event "Command Selection": Double Click {
        n250 = event-data() -> ("Row"=w414:i32)  [unwired: 1 in]
        n251 = property on="Command Selection" class="MCListbox (strict)"() -> ("ItemNames"=w417:string[][])  [unwired: 2 in, 2 out]
        n252 = local read "Command Params"() -> (w413:string[][])
        n253 = Index Array(array=w417, index (row)=w414, index (col)=0) -> (element=w415:string)
        n254 = call <vilib>:"Invoke Commands.vi"("Command Params"=w413, "Function Name"=w415) -> ("Params"=w412:u8, "Started"=w407:bool)  [unwired: 7 in, 1 out]
        n255 = Array Subset(array=w413, length (row)=w412) -> (w411:string[][])  [unwired: 3 in]
        n256 = Select(t="Executing" ("Cmd Status"), s=w407, f="" ("Cmd Status")) -> (s? t:f=w408:string)
        n257 = local write "Cmd Status"(w408) -> ()
      }
      event "CheckList": Double Click {
        # "Shift clears all"
        # "Update symbols on the listbox"
        n258 = event-data() -> ("PlatMods.Shift"=w419:bool, "Row"=w421:i32)  [unwired: 1 in]
        n259 = case shown="True" w419 {
          tunnel: w421 -> [w425 _]
          tunnel: 1 -> [w424 _]
          frame False {
            n260 = property on="CheckList" class="LstBox (strict)"() -> ("Item Symbols"=w423:i32[])  [unwired: 2 in, 2 out]
            n261 = Replace Array Subset(array=w423, new element=w424, index=w425) -> (w422:i32[])
            n262 = property on="CheckList" class="LstBox (strict)"("Item Symbols"=w422) -> ()  [unwired: 2 in, 2 out]
          }
          frame True {
            w426 = 0 ("Top Row")
            n263 = property on="CheckList" class="LstBox (strict)"() -> ("Number of Rows"=w428:u32)  [unwired: 2 in, 2 out]
            n264 = Initialize Array(0, w428) -> (w427:i32[])
            n265 = property on="CheckList" class="LstBox (strict)"("Top Row"=w426, "Value"=w426, "Item Symbols"=w427) -> ()  [unwired: 2 in, 2 out]
          }
        }
      }
      event "CheckList": Key Down {
        # "Update symbols on the listbox\nLeft and right keys check and uncheck"
        n266 = event-data() -> ("VKey"=w432:T21)  [unwired: 1 in]
        n267 = case shown="\"Left\", \"Right\"" w432 {
          selector: w432 -> [w437 _]
          tunnel: eventvkey."Left" ("VKey") -> [w435 _]
          frame "Left", "Right" {
            n268 = Equal?(x=w435, y=w437) -> (x = y?=w436:bool)
            n269 = Select(t=0, s=w436, f=1) -> (s? t:f=w438:i32)
            n270 = property on="CheckList" class="LstBox (strict)"() -> ("Item Symbols"=w441:i32[])  [unwired: 2 in, 2 out]
            n271 = Replace Array Subset(array=w441, new element=w438, index="CheckList") -> (w440:i32[])
            n272 = property on="CheckList" class="LstBox (strict)"("Item Symbols"=w440) -> ()  [unwired: 2 in, 2 out]
          }
          frame Default {
          }
        }
      }
      event "Motor.Enable": Value Change {
        # "When the test mode otor enable helper is set, update that\ntree row item's value"
        n273 = event-data() -> ("NewVal"=w447:bool)  [unwired: 1 in]
        n274 = Unbundle("Motor") -> ("Value"=w446:dbl)  [unwired: 1 out]
        n275 = Select(t=w446, s=w447, f=0.0) -> (s? t:f=w444:dbl)
        n276 = call <vilib>:"NT Write Number.vi"("Numeric"=w444, "Name"=w443) -> ()  [unwired: 9 in, 1 out]
      }
      event "Test Slider": Value Change {
        # "When the test mode slider helper is set, update that\ntree row item's value"
        n277 = event-data() -> ("NewVal"=w450:dbl)  [unwired: 1 in]
        n278 = call <vilib>:"NT Write Number.vi"("Numeric"=w450, "Name"=w451) -> ()  [unwired: 9 in, 1 out]
      }
      event "On/Off": Value Change {
        # "When the test mode on/off helper value is set, update that\ntree row item's value"
        n279 = event-data() -> ("NewVal"=w455:bool)  [unwired: 1 in]
        n280 = Boolean To (0,1)(Boolean=w455) -> (0, 1=w454:i16)
        n281 = call <vilib>:"NT Write Number.vi"("Numeric"=w454, "Name"=w453) -> ()  [unwired: 9 in, 1 out]
      }
      event "Rev/Fwd": Value Change {
        # "When the test mode helper value for relays is set, update that\ntree row item's value"
        n282 = event-data() -> ("NewVal.Forward"=w463:bool, "NewVal.Reverse"=w462:bool)  [unwired: 1 in]
        n283 = Boolean To (0,1)(Boolean=w463) -> (0, 1=w459:i16)
        n284 = Boolean To (0,1)(Boolean=w462) -> (0, 1=w461:i16)
        n285 = Negate(x=w461) -> (-x=w460:i16)
        n286 = Add(x=w459, y=w460) -> (x+y=w458:i16)
        n287 = call <vilib>:"NT Write Number.vi"("Numeric"=w458, "Name"=w457) -> ()  [unwired: 9 in, 1 out]
      }
      event "Test Ring": Value Change {
        # "When a test mode helper value is selected from the ring,\nset the tree item's variable to the string value"
        n288 = event-data() -> ("NewVal"=w467:u16)  [unwired: 1 in]
        n289 = property on="Test Ring" class="Ring (strict)"() -> ("Strings []"=w468:string[])  [unwired: 2 in, 2 out]
        n290 = Index Array(array=w468, index=w467) -> (element=w466:string)
        n291 = call <vilib>:"NT Write String.vi"("String"=w466, "Name"=w465) -> ()  [unwired: 9 in, 1 out]
      }
      event "Rec Mode": Value Change {
        # "Update globals for recording mode and path to read log from.\nClear when logging and let NetworkTables set path for vision to\nuse."
        n292 = event-data() -> ("NewVal"=w479:enum32{"Stop", "Record", "Playback"})  [unwired: 1 in]
        n293 = global write "WPI_DashboardLogging Global.vi" "Logging Filename"(path "") -> ()
        n294 = global write "WPI_DashboardLogging Global.vi" "Recording"(w479) -> ()
        n295 = case shown="\"Playback\"" w479 {
          tunnel: w478 -> [_ w481 w490]
          tunnel: [_ _ w489] -> w476
          tunnel: [_ _ w488] -> _
          tunnel: w474 -> [_ _ w486]
          tunnel: cluster{i32, i32} {-250, 170} -> [_ _ w485]
          tunnel: [_ _ T22 {"Image Size"=TRUE, "Image Type"=TRUE, "Pixel Value"=TRUE, "ROI Information"=TRUE, "Zoom Factor"=FALSE} ("Image Information Shown:All Elements")] -> w469
          tunnel: [_ _ TRUE ("Zoom Factor")] -> w470
          tunnel: w472 -> [_ _ w482]
          frame Default {
          }
          frame "Stop", "Record" {
            # "Place Window too"
            n296 = invoke class="VI" method="FP.Close"(reference=w481) -> (reference out=w480:refnum<vi>)  [unwired: 2 in, 2 out]
            n297 = invoke class="VI" method="Abort VI"(reference=w480) -> ()  [unwired: 2 in, 3 out]
          }
          frame "Playback" {
            n298 = call "Open Playback Panel.vi"("Offset"=w485, "DB VI Ref"=w486, "Playback in"=w490) -> ("Playback out"=w487:refnum<vi>)  [unwired: 8 in]
            n299 = register-events(w487, w482) -> (reference out=w489:refnum<event-registration>, error out=w488:errorcluster)  [unwired: 2 in]
          }
        }
        n300 = property on="Camera Image Right" class="ImageControl"("Image Information Shown"=w469, "Image Information Visible"=w470) -> ()  [unwired: 2 in, 2 out]
        n301 = property on="Camera Image" class="ImageControl"("Image Information Shown"=w469, "Image Information Visible"=w470) -> ()  [unwired: 2 in, 2 out]
        n302 = call <vilib>:"WPI_DashboardNT Log FieldName Cache.vi"("Operation"=enum16{"Lookup/Add", "Index", "Clear"}."Clear") -> ()  [unwired: 8 in, 3 out]
      }
      event Panel Close {
        w492 = enum32{"Stop", "Record", "Playback"}."Stop" ("Rec Mode")
        # "Playback window has been closed, abort"
        n303 = event-data() -> ()  [unwired: 1 in, 4 out]
        n304 = local write "Rec Mode"(w492) -> ()
        n305 = global write "WPI_DashboardLogging Global.vi" "Recording"(w492) -> ()
      }
      event Panel Close {
        # "Abort playback window and ourself"
        n306 = event-data() -> ()  [unwired: 1 in, 4 out]
        n307 = invoke class="VI" method="FP.Close"(reference=w496) -> (reference out=w495:refnum<vi>)  [unwired: 2 in, 2 out]
        n308 = invoke class="VI" method="Abort VI"(reference=w495) -> (error out=w494:errorcluster)  [unwired: 2 in, 2 out]
        n309 = invoke class="VI" method="Abort VI"(error in=w494) -> ()  [unwired: 2 in, 3 out]
      }
      event User Event {
        n310 = event-data() -> ("IDs"=w503:cluster{"RPC field ID":u16, "Unique ID":u16}, "String"=w502:string)  [unwired: 1 in]
        n311 = Bundle("IDs"=w503, "String"=w502) -> (w501:T9)  [unwired: 1 in]
        n312 = call <vilib>:"Retrieve RPC Response.vi"("RPC Response"=w501) -> ("Output"=w499:string[][])  [unwired: 10 in]
        n313 = Build Array (concatenate)(w497, w499) -> (w498:string[][])
        n314 = local write "Command Params"(w498) -> ()
        n315 = local write "Cmd Status"("" ("Cmd Status")) -> ()
      }
      event "Tree": Double Click {
        n316 = event-data() -> ("PlatMods"=w509:T25, "Tag"=w506:string)  [unwired: 1 in]
        n317 = Unbundle(w509) -> ("Shift"=w508:bool)  [unwired: 4 out]
        n318 = String Subset(string=w506, length (rest)=1 ("length (rest)")) -> (substring=w505:string)  [unwired: 1 in]
        n319 = Not(x=w508) -> (.not. x?=w507:bool)
        n320 = case shown="\"/\"" w505 {
          tunnel: w506 -> [_ w512]
          tunnel: w507 -> [_ w511]
          frame Default {
          }
          frame "/" {
            n321 = call <vilib>:"NT Update Persistence.vi"("Persistence"=w511, "Name"=w512) -> ()  [unwired: 9 in, 1 out]
          }
        }
      }
    }
  }
  n322 = while {
    tunnel: w65 -> [w514]
    i -> [w517]
    stop <- FALSE stop-if-true
    n323 = Wait (ms)(milliseconds to wait=u32 100) -> ()  [unwired: 1 out]
    n324 = case shown="\"Playback\"" "Rec Mode" {
      tunnel: w517 -> [_ _ w532]
      tunnel: [u32 2829099 ("Base Color") u32 11141120 ("Target Color") w521] -> w513
      frame "Stop", Default {
        # "Reset the color, extra updates don't cost much"
      }
      frame "Record" {
      }
      frame "Playback" {
        # "Playback"
        n325 = Quotient & Remainder(x=w532, y=u32 50 ("milliseconds to wait")) -> (x-y*floor(x/y)=w528:u32)  [unwired: 1 out]
        n326 = Divide(x=w528, y=u32 50 ("milliseconds to wait")) -> (x/y=w525:dbl)
        n327 = Multiply(x=6.283185307179586, y=w525) -> (x*y=w530:dbl)
        n328 = Sine(x=w530) -> (sin(x)=w529:dbl)
        n329 = Absolute Value(x=w529) -> (abs(x)=w522:dbl)
        n330 = call "Interpolate RGB Color.vi"("Proportion"=w522, "Target Color"=u32 30976, "Base Color"=u32 2829099) -> ("Result Color"=w521:u32)  [unwired: 8 in]
      }
    }
    n331 = property class="Pane"(reference=w514, "PaneColor"=w513) -> ()  [unwired: 1 in, 2 out]
  }
  n332 = local write "Dashboard Tab"(T2."Drive" ("Dashboard Tab")) -> ()
  n333 = property on="On/Off" class="Bool (strict)"("Visible"=w37) -> ()  [unwired: 2 in, 2 out]
  n334 = property on="Motor" class="Clust (strict)"("Visible"=w37) -> ()  [unwired: 2 in, 2 out]
  n335 = property on="Progress" class="Clust (strict)"("Visible"=w37) -> ()  [unwired: 2 in, 2 out]
  n336 = property on="Test Ring" class="Ring (strict)"("Visible"=w37) -> ()  [unwired: 2 in, 2 out]
  n337 = property on="Rev/Fwd" class="Clust (strict)"("Visible"=w37) -> ()  [unwired: 2 in, 2 out]
  n338 = while {
    tunnel: u16 1741 ("timeout ms (25000)") -> [w534]
    stop <- FALSE stop-if-true
    n339 = TCP Create Listener(10:w534) -> (0:w533:errorcluster, 3:w535:refnum<k5>)  [unwired: 4 in, 1 out]
    n340 = case shown="No Error" w533 {
      selector: w533 -> [w537 _]
      tunnel: w535 -> [w538 _]
      frame No Error {
        n341 = while {
          tunnel: w538 -> [w541]
          tunnel: w537 -> [w540]
          stop <- FALSE stop-if-true
          n342 = TCP Wait On Listener(8:w540, 11:w541) -> (0:w542:errorcluster, 4:w543:refnum<k5>)  [unwired: 2 in, 3 out]
          n343 = local write "TCP"(w543) -> ()
          n344 = case shown="No Error" w542 {
            frame No Error {
            }
            frame Error {
              n345 = Wait (ms)(milliseconds to wait=u32 1000) -> ()  [unwired: 1 out]
            }
          }
        }
      }
      frame Error {
        n346 = Wait (ms)(milliseconds to wait=u32 1000) -> ()  [unwired: 1 out]
      }
    }
  }
  n347 = local write "Command Selection"(u16 0 ("milliseconds to wait")) -> ()
  n348 = local write "Command Params"(string[][] [] ("Command Params")) -> ()
  n349 = global write "WPI_DashboardLogging Global.vi" "Recording"(w59) -> ()
  n350 = local write "Rec Mode"(w59) -> ()
  n351 = call <vilib>:"NT Write String.vi"("String"="Select Auto", "Name"="Auto Selector") -> ()  [unwired: 9 in, 1 out]
